vi "-8000 Unspecified Error--error.vi"(8 "error in":errorcluster, 11 "Argument":string) -> (0 "error out":errorcluster, 2 "Error Code":i32)   [LabVIEW 2020, in "PCANBasic.lvlib"]
uses:
  PCANBasic.lvlib
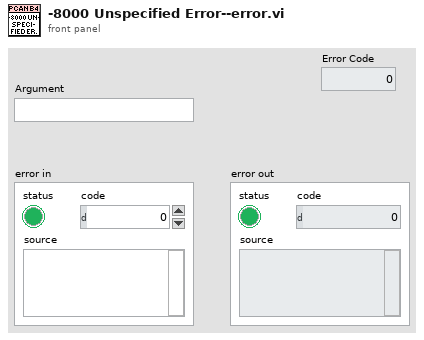
[diagram p1: front panel]
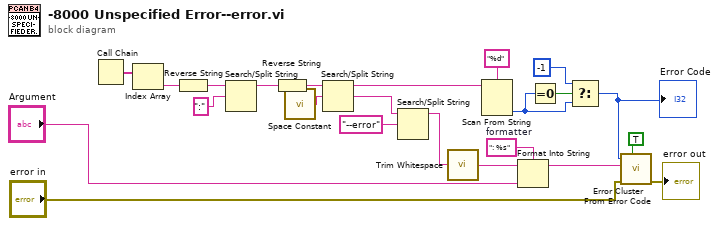
[diagram p0: block diagram]
diagram:
  w20 = ": %s"  # formatter
  n1 = Call Chain() -> (call chain=w12:string[])
  n2 = Index Array(array=w12) -> (element=w6:string)  [unwired: 1 in]
  n3 = Reverse String(1:w6) -> (0:w11:string)
  n4 = Search/Split String(string=w11, search string/char (-)=":") -> (substring before match=w10:string)  [unwired: 1 in, 2 out]
  n5 = Reverse String(1:w10) -> (0:w8:string)
  n6 = call <vilib>:"Space Constant.vi"() -> ("String"=w7:string)
  n7 = Search/Split String(string=w8, search string/char (-)=w7) -> (substring before match=w5:string, match + rest of string=w3:string)  [unwired: 1 in, 1 out]
  n8 = Search/Split String(string=w3, search string/char (-)="--error") -> (substring before match=w2:string)  [unwired: 1 in, 2 out]
  n9 = call <vilib>:"Trim Whitespace.vi"("string"=w2) -> ("trimmed string"=w1:string)  [unwired: 1 in]
  n10 = Scan From String(format string="%d", input string=w5) -> (output 1=w16:i32)  [unwired: 3 in, 3 out]
  n11 = Format Into String(format string=w20, initial string=w1, "Argument") -> (resulting string=w21:string)  [unwired: 1 in, 1 out]
  n12 = Equal To 0?(x=w16) -> (x = 0?=w17:bool)
  n13 = Select(t=-1, s=w17, f=w16) -> (s? t:f=w14:i32)
  "Error Code" <- w14
  n14 = call <vilib>:"Error Cluster From Error Code.vi"("show call chain? (False)"=TRUE, "error in (no error)"="error in", "error message (\"\")"=w21, "error code (0)"=w14) -> ("error out"=→"error out":errorcluster)  [unwired: 5 in]
